vi "Set Thermostat Target Temperature.vi"   [LabVIEW 2013, in "LMH-Nest.lvlib"]
doc: "Set the Nest device target temperature."
uses:
  LMH-Nest.lvlib
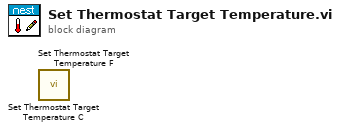
[diagram p0: block diagram]
diagram:
  n1 = call "Set Thermostat Target Temperature C.vi"() -> ()  [unwired: 10 in, 2 out]
  n2 = call "Set Thermostat Target Temperature F.vi"() -> ()  [unwired: 10 in, 2 out]
